vi "example_2_6_b.vi"() -> ()   [LabVIEW 2018]
panel:
  in  "ADD/SUB":bool
  in  "Numeric 3":dbl format="%.2f"
  out "Numeric 2":dbl format="%.2f"
  in  "Numeric":dbl format="%.2f"
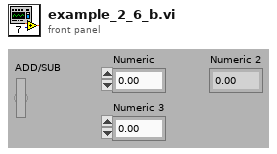
[diagram p1: front panel]
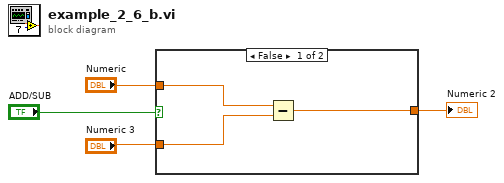
[diagram p0: block diagram]
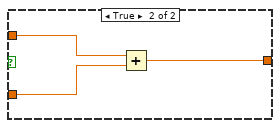
[diagram p2: hidden frame]
diagram:
  n1 = case shown="False" "ADD/SUB" {
    tunnel: "Numeric" -> [w6 w10]
    tunnel: "Numeric 3" -> [w5 w9]
    tunnel: [w7 w8] -> w1
    frame False {
      n2 = Subtract(x=w6, y=w5) -> (x-y=w7:dbl)
    }
    frame True {
      n3 = Add(x=w10, y=w9) -> (x+y=w8:dbl)
    }
  }
  "Numeric 2" <- w1
